vi "Parameters_BuildReference.vi"(11 "Reference Move Parameters":T1={"Reference Move Mode"=3, "Start Search Forward"=FALSE, "Stop on FWD Edge"=FALSE, "Approach Forward"=FALSE, "Velocity"=0.0, "Acceleration"=0.0}) -> (3 "Parameters":dbl[](array[numeric]))   [LabVIEW 2017, in "WordManipulationLibrary.lvlib"]
uses:
  WordManipulationLibrary.lvlib
  ReferenceMoveParameters.ctl
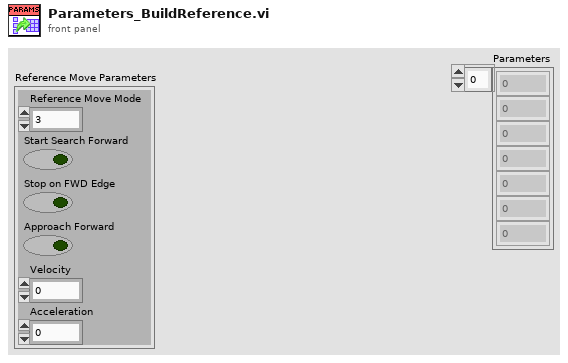
[diagram p1: front panel]
types:
  T1 = typedef "WordManipulationLibrary.lvlib/ReferenceMoveParameters.ctl" = cluster{"Reference Move Mode":i32, "Start Search Forward":bool, "Stop on FWD Edge":bool, "Approach Forward":bool, "Velocity":dbl, "Acceleration":dbl}
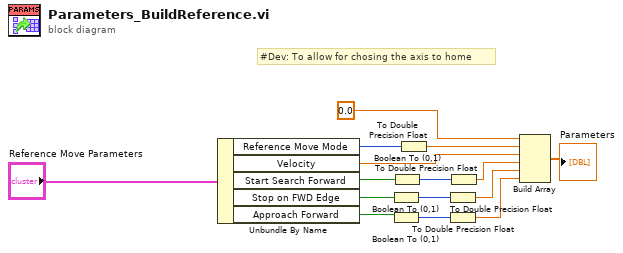
[diagram p0: block diagram]
diagram:
  # "#Dev: To allow for chosing the axis to home"
  n1 = Unbundle By Name("Reference Move Parameters") -> ("Reference Move Mode"=w14:i32, "Velocity"=w12:dbl, "Start Search Forward"=w11:bool, "Stop on FWD Edge"=w7:bool, "Approach Forward"=w6:bool)
  n2 = Boolean To (0,1)(Boolean=w7) -> (0, 1=w9:i16)
  n3 = Boolean To (0,1)(Boolean=w6) -> (0, 1=w8:i16)
  n4 = Boolean To (0,1)(Boolean=w11) -> (0, 1=w10:i16)
  n5 = To Double Precision Float(number=w14) -> (double precision float=w13:dbl)
  n6 = To Double Precision Float(number=w9) -> (double precision float=w4:dbl)
  n7 = To Double Precision Float(number=w8) -> (double precision float=w3:dbl)
  n8 = To Double Precision Float(number=w10) -> (double precision float=w5:dbl)
  n9 = Build Array(0.0 ("element"), w13, w12, w5, w4, w3) -> (→"Parameters":dbl[])
